vi "ErrorCheckHWI.vi"(8 "error in (no error)":errorcluster, 11 "TestMenu in":refnum<class "TestMenu.lvclass">) -> (0 "error out":errorcluster, 3 "TestMenu out":refnum<class "TestMenu.lvclass">)   [LabVIEW 2013, in "TestMenu.lvclass"]
uses:
  TestMenu.lvclass
  Device/Device.lvclass
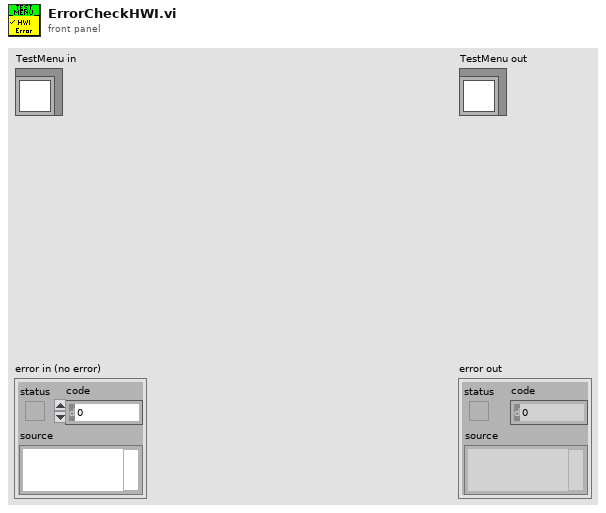
[diagram p1: front panel]
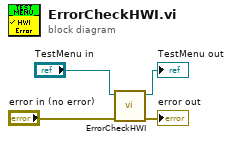
[diagram p0: block diagram]
diagram:
  n1 = call-parent "ErrorCheckHWI.vi"("error in (no error)"="error in (no error)", "Device in"="TestMenu in") -> ("error out"=→"error out":errorcluster, "Device out"=→"TestMenu out":refnum<class "TestMenu.lvclass">)  [unwired: 8 in]
